vi "SENS_FOM_DISP_SEL.vi"(0 "VISA IN":refnum<visa-resource-name>, 1 "Frq. Range Name":string, 5 "error in":errorcluster, 7 "Channel":i32) -> (14 "VISA Out":refnum<visa-resource-name>, 19 "error out":errorcluster)   [LabVIEW 2018, in "PNA-X.lvlib"]
doc: "SENSe<cnum>:FOM:DISPlay:SELect <string> \n(Read-Write) Select the range to be displayed on the PNA x-axis. All traces in the channel have this same x-axis \nscaling. \nParameters \n<cnum> Any existing channel number; if unspecified, value is set to 1. \n<string> Range name. Case insensitive. Use SENSe:FOM:CAT? to see a list of available \nfrequency range names. \nExamples SENS:FOM:DISPlay:SELect \"source2\" \nsense2:fom:display:select \"source\" \nQuery Syntax SENSe<cnum>:FOM:DISPlay:SELect? \nReturn Type String \nDefault Receivers"
uses:
  PNA-X.lvlib
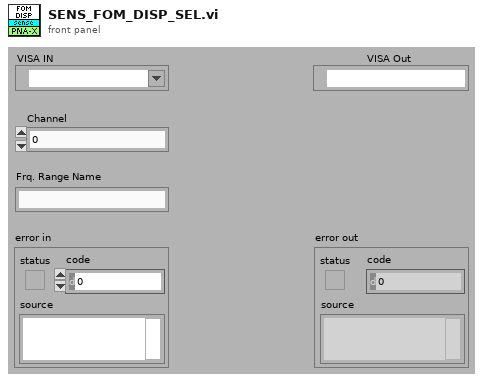
[diagram p1: front panel]
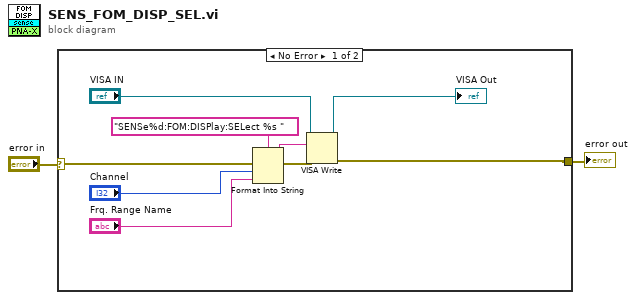
[diagram p0: block diagram]
diagram:
  n1 = case shown="No Error" "error in" {
    selector: "error in" -> [w11 w12]
    tunnel: [w6 w12] -> w1
    frame No Error {
      n2 = Format Into String(format string="SENSe%d:FOM:DISPlay:SELect %s " ("Cmdline"), error in=w11, "Channel", "Frq. Range Name") -> (resulting string=w9:string, error out=w10:errorcluster)  [unwired: 1 in]
      n3 = VISA Write(VISA resource name="VISA IN", write buffer=w9, error in (no error)=w10) -> (VISA resource name out=→"VISA Out":refnum<visa-resource-name>, error out=w6:errorcluster)  [unwired: 1 out]
    }
    frame Error {
    }
  }
  "error out" <- w1
